vi "arrayrng.vi"(4 "barrier?":bool, 5 "mine count":i32, 6 "sizeoffset":i32, 7 "empty array":i8[][][](array[numeric]), 9 "size":i32, 10 "layers":i32, 11 "barrier count":i32) -> (3 "Array out":i8[][][](array[numeric]))   [LabVIEW 2025]
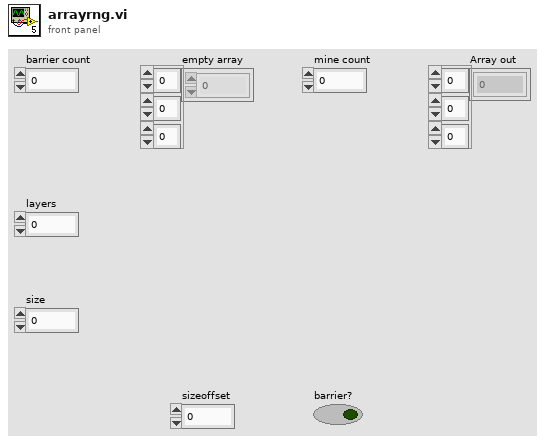
[diagram p1: front panel]
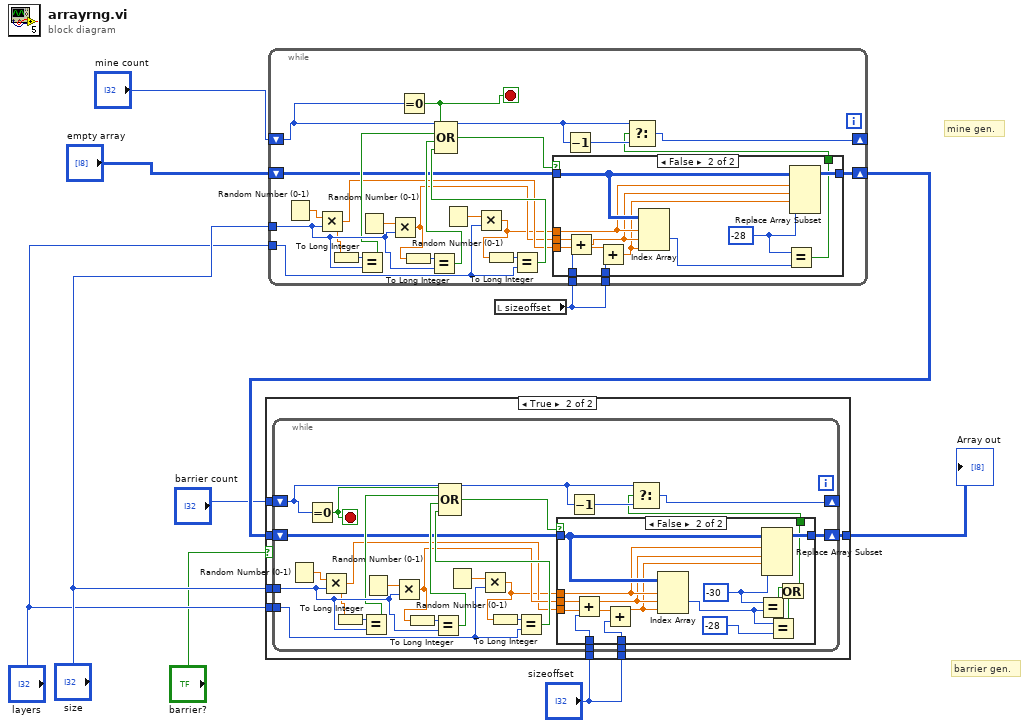
[diagram p0: block diagram]
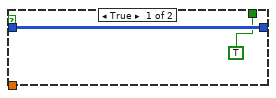
[diagram p3: hidden frame]
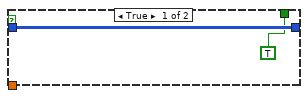
[diagram p4: hidden frame]
diagram:
  # "barrier gen."
  # "mine gen."
  n1 = local read "sizeoffset"() -> (w1:i32)
  n2 = while {
    shift-right: [w34] -> w6
    shift-left: "empty array" -> [w22]
    tunnel: "layers" -> [w23]
    tunnel: "size" -> [w29]
    shift-right: [w16] -> _
    shift-left: "mine count" -> [w14]
    tunnel: w1 -> [w13]
    tunnel: w1 -> [w12]
    stop <- w11 stop-if-true
    n3 = Random Number (0-1)() -> (number: 0 to 1=w33:dbl)
    n4 = Multiply(x=w33, y=w29) -> (x*y=w21:dbl)
    n5 = To Long Integer(number=w21) -> (32bit integer=w31:i32)
    n6 = Equal?(x=w31, y=w29) -> (x = y?=w26:bool)
    n7 = Random Number (0-1)() -> (number: 0 to 1=w32:dbl)
    n8 = Multiply(x=w32, y=w29) -> (x*y=w20:dbl)
    n9 = Equal To 0?(x=w14) -> (x = 0?=w11:bool)
    n10 = To Long Integer(number=w20) -> (32bit integer=w30:i32)
    n11 = Equal?(x=w30, y=w29) -> (x = y?=w25:bool)
    n12 = Random Number (0-1)() -> (number: 0 to 1=w27:dbl)
    n13 = Multiply(x=w27, y=w23) -> (x*y=w19:dbl)
    n14 = To Long Integer(number=w19) -> (32bit integer=w28:i32)
    n15 = Equal?(x=w28, y=w23) -> (x = y?=w24:bool)
    n16 = Compound Arithmetic op=OR(w11, w26, w25, w24) -> (w18:bool)
    n17 = case shown="False" w18 {
      tunnel: [w36 w48] -> w34
      tunnel: w22 -> [w36 w47]
      tunnel: w21 -> [_ w39]
      tunnel: w20 -> [_ w42]
      tunnel: w19 -> [_ w43]
      tunnel: [TRUE w44] -> w15
      tunnel: w13 -> [_ w40]
      tunnel: w12 -> [_ w37]
      frame True {
      }
      frame False {
        w45 = i8 -28 ("element")
        n18 = Add(x=w42, y=w40) -> (x+y=w41:dbl)
        n19 = Add(x=w39, y=w37) -> (x+y=w38:dbl)
        n20 = Index Array(array=w47, index (dim 0)=w43, index (dim 1)=w41, index (dim 2)=w38) -> (element=w46:i8)
        n21 = Equal?(x=w45, y=w46) -> (x = y?=w44:bool)
        n22 = Replace Array Subset(array=w47, new element=w45, index (dim 0)=w43, index (dim 1)=w41, index (dim 2)=w38) -> (w48:i8[][][])
      }
    }
    n23 = Decrement(x=w14) -> (x-1=w17:i32)
    n24 = Select(t=w14, s=w15, f=w17) -> (s? t:f=w16:i32)
  }
  n25 = case shown="True" "barrier?" {
    tunnel: "size" -> [_ w56]
    tunnel: "layers" -> [_ w55]
    tunnel: "barrier count" -> [_ w54]
    tunnel: w6 -> [w49 w53]
    tunnel: [w49 w52] -> w8
    tunnel: "sizeoffset" -> [_ w51]
    tunnel: "sizeoffset" -> [_ w50]
    frame False {
    }
    frame True {
      n26 = while {
        shift-right: [w80] -> w52
        shift-left: w53 -> [w68]
        tunnel: w55 -> [w69]
        tunnel: w56 -> [w75]
        shift-right: [w64] -> _
        shift-left: w54 -> [w62]
        tunnel: w51 -> [w59]
        tunnel: w50 -> [w58]
        stop <- w57 stop-if-true
        n27 = Random Number (0-1)() -> (number: 0 to 1=w79:dbl)
        n28 = Equal To 0?(x=w62) -> (x = 0?=w57:bool)
        n29 = Multiply(x=w79, y=w75) -> (x*y=w61:dbl)
        n30 = To Long Integer(number=w61) -> (32bit integer=w77:i32)
        n31 = Equal?(x=w77, y=w75) -> (x = y?=w72:bool)
        n32 = Random Number (0-1)() -> (number: 0 to 1=w78:dbl)
        n33 = Multiply(x=w78, y=w75) -> (x*y=w67:dbl)
        n34 = To Long Integer(number=w67) -> (32bit integer=w76:i32)
        n35 = Equal?(x=w76, y=w75) -> (x = y?=w71:bool)
        n36 = Random Number (0-1)() -> (number: 0 to 1=w73:dbl)
        n37 = Multiply(x=w73, y=w69) -> (x*y=w60:dbl)
        n38 = To Long Integer(number=w60) -> (32bit integer=w74:i32)
        n39 = Equal?(x=w74, y=w69) -> (x = y?=w70:bool)
        n40 = Compound Arithmetic op=OR(w57, w72, w71, w70) -> (w66:bool)
        n41 = case shown="False" w66 {
          tunnel: [w82 w97] -> w80
          tunnel: w68 -> [w82 w96]
          tunnel: w60 -> [_ w94]
          tunnel: w67 -> [_ w88]
          tunnel: w61 -> [_ w86]
          tunnel: [TRUE w90] -> w63
          tunnel: w59 -> [_ w83]
          tunnel: w58 -> [_ w85]
          frame True {
          }
          frame False {
            w95 = i8 -30 ("element")
            n42 = Add(x=w88, y=w83) -> (x+y=w87:dbl)
            n43 = Add(x=w86, y=w85) -> (x+y=w84:dbl)
            n44 = Index Array(array=w96, index (dim 0)=w94, index (dim 1)=w87, index (dim 2)=w84) -> (element=w93:i8)
            n45 = Equal?(x=w95, y=w93) -> (x = y?=w92:bool)
            n46 = Replace Array Subset(array=w96, new element=w95, index (dim 0)=w94, index (dim 1)=w87, index (dim 2)=w84) -> (w97:i8[][][])
            n47 = Equal?(x=w93, y=i8 -28 ("element")) -> (x = y?=w91:bool)
            n48 = Or(x=w92, y=w91) -> (x .or. y?=w90:bool)
          }
        }
        n49 = Decrement(x=w62) -> (x-1=w65:i32)
        n50 = Select(t=w62, s=w63, f=w65) -> (s? t:f=w64:i32)
      }
    }
  }
  "Array out" <- w8
